vi "RunScanMessage.vi"() -> (3 "RunScanMessage":string)   [LabVIEW 2019]
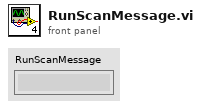
[diagram p1: front panel]
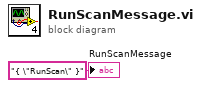
[diagram p0: block diagram]
diagram:
  "RunScanMessage" <- "{ \"RunScan\" }" ("RunScanMessage")
